vi "Fixed-Point Raw to Double.vi"(1 "Signed?":bool=TRUE, 2 "Word Length":u8, 3 "Data":bool[](array[boolean]), 4 "Delta":dbl format="%#_13g") -> (0 "value":dbl)   [LabVIEW 2018]
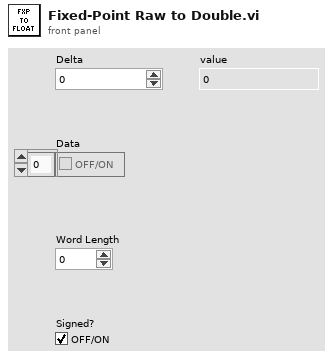
[diagram p1: front panel]
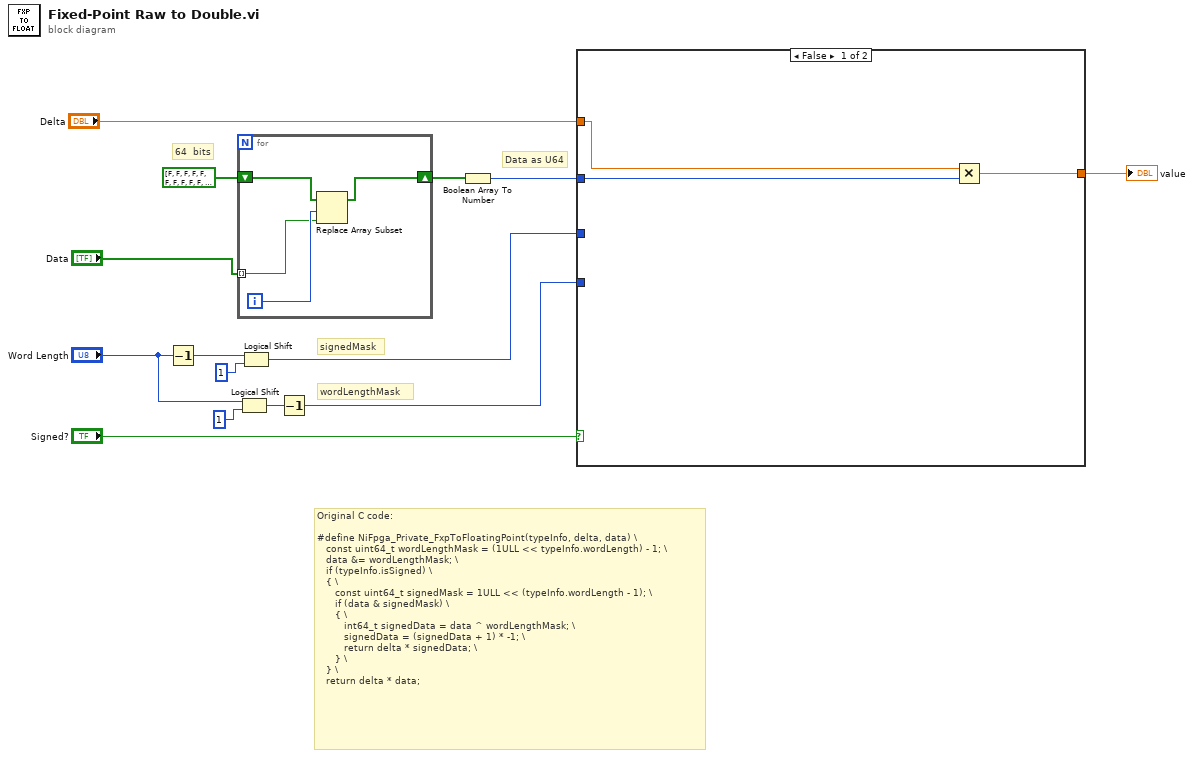
[diagram p0: block diagram]
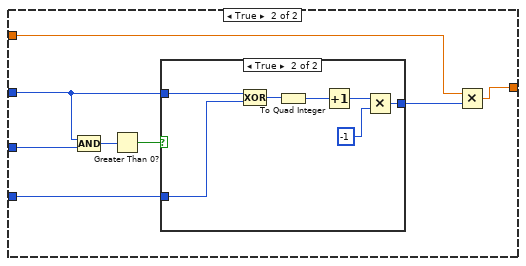
[diagram p2: hidden frame]
diagram:
  # "Original C code: \n\n#define NiFpga_Private_FxpToFloatingPoint(typeInfo, delta, data) \\\n   const uint64_t wordLengthMask = (1ULL << typeInfo.wordLength) - 1; \\\n   data &= wordLengthMask; \\\n   if (typeInfo.isSigned) \\\n   { \\\n      const uint64_t signedMask = 1ULL << (typeInfo.wordLength - 1); \\\n      if (data & signedMask) \\\n      { \\\n         int64_t signedData = data ^ wordLengthMask; \\\n         signedData = (signedData + 1) * -1; \\\n         return delta * signedData; \\\n      } \\\n   } \\\n   return delta * data;"
  # "wordLengthMask"
  # "signedMask"
  # "Data as U64"
  # "64  bits"
  n1 = Decrement(x="Word Length") -> (x-1=w9:u8)
  n2 = for {
    shift-right: [w17] -> w12
    shift-left: bool[] [FALSE, FALSE, FALSE, FALSE, FALSE, FALSE, FALSE, FALSE, FALSE, FALSE, FALSE, FALSE, FALSE, FALSE, FALSE, FALSE, FALSE, FALSE, FALSE, FALSE, FALSE, FALSE, FALSE, FALSE, FALSE, FALSE, FALSE, FALSE, FALSE, FALSE, FALSE, FALSE, FALSE, FALSE, FALSE, FALSE, FALSE, FALSE, FALSE, FALSE, FALSE, FALSE, FALSE, FALSE, FALSE, FALSE, FALSE, FALSE, FALSE, FALSE, FALSE, FALSE, FALSE, FALSE, FALSE, FALSE, FALSE, FALSE, FALSE, FALSE, FALSE, FALSE, FALSE, FALSE] -> [w18]
    tunnel: "Data" -> [w15] mode=indexing
    i -> [w16]
    n3 = Replace Array Subset(array=w18, new element=w15, index=w16) -> (w17:bool[])
  }
  n4 = Logical Shift(y="Word Length", x=u64 1) -> (x << y=w5:u64)
  n5 = Logical Shift(y=w9, x=u64 1) -> (x << y=w8:u64)
  n6 = Decrement(x=w5) -> (x-1=w4:u64)
  n7 = Boolean Array To Number(Boolean array=w12) -> (number=w10:u64)
  n8 = case shown="False" "Signed?" {
    tunnel: w10 -> [w20 w26]
    tunnel: w8 -> [_ w29]
    tunnel: w4 -> [_ w25]
    tunnel: "Delta" -> [w21 w24]
    tunnel: [w19 w22] -> w1
    frame False {
      n9 = Multiply(x=w21, y=w20) -> (x*y=w19:dbl)
    }
    frame True {
      n10 = Compound Arithmetic op=AND(w26, w29) -> (w28:u64)
      n11 = Greater Than 0?(x=w28) -> (x > 0?=w27:bool)
      n12 = case shown="True" w27 {
        tunnel: w26 -> [_ w36]
        tunnel: w25 -> [_ w35]
        tunnel: [_ w30] -> w23
        frame False {
        }
        frame True {
          n13 = Compound Arithmetic op=XOR(w36, w35) -> (w34:u64)
          n14 = To Quad Integer(1:w34) -> (0:w33:i64)
          n15 = Increment(x=w33) -> (x+1=w32:i64)
          n16 = Multiply(x=w32, y=i64 -1) -> (x*y=w30:i64)
        }
      }
      n17 = Multiply(x=w24, y=w23) -> (x*y=w22:dbl)
    }
  }
  "value" <- w1
